vi "Write.vi"(8 "error in (no error)":errorcluster, 10 "Value":T1, 11 "Double Float.lvclass_340760 in":refnum<class "Var_CPLX_EXT.lvclass">) -> (0 "error out":errorcluster, 3 "Double Float.lvclass_340760 out":refnum<class "Var_CPLX_EXT.lvclass">)   [LabVIEW 2021, in "Var_CPLX_EXT.lvclass"]
uses:
  Var_CPLX_EXT.lvclass
  Type.ctl
  Var_CPLX_EXT.lvclass/Var_CPLX_EXT.ctl
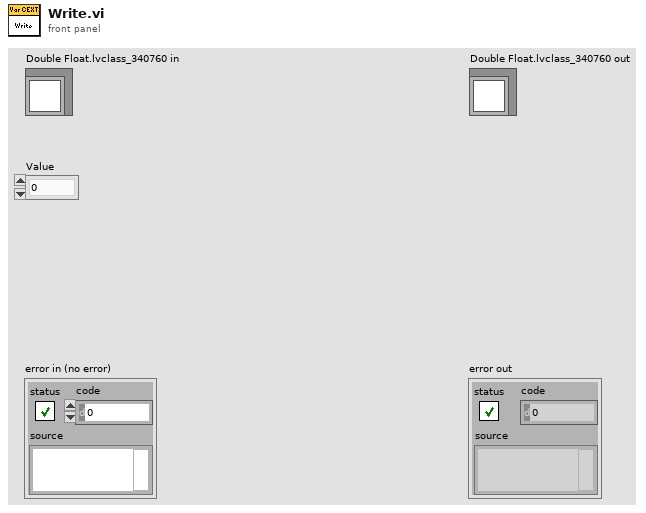
[diagram p1: front panel]
types:
  T1 = typedef "Var_CPLX_EXT.lvclass/Type.ctl" = cxt
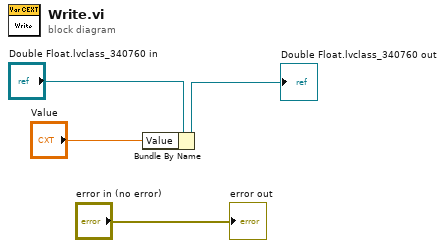
[diagram p0: block diagram]
diagram:
  n1 = Bundle By Name(cluster="Double Float.lvclass_340760 in", "Value"="Value") -> (→"Double Float.lvclass_340760 out":refnum<class "Var_CPLX_EXT.lvclass">)
  "error out" <- "error in (no error)"
